vi "Client Single Connection.vi"() -> ()   [LabVIEW 2020]
doc: "This WebSockets API example VI acts as a client to make an outgoing websockets connection. Receives/sends string data to the connected server.\nWebSockets 2.0.1.40\nSam Sharp - MediaMongrels Ltd\nCopyright (c) 2019, MediaMongrels Ltd"
uses:
  Libraries/RPI.SenseHat.Joystick/TypeDefs/Joystick.ctl
  <vilib>/MediaMongrels Ltd/WebSockets/WebSockets/WebSocket/WebSocket.lvclass/WebSocket.ctl
  <vilib>/MediaMongrels Ltd/WebSockets/WebSockets/WebSocket Client/WebSocket Client.lvclass
  C:/Program Files (x86)/National Instruments/LabVIEW 2020/vi.lib/MediaMongrels Ltd/WebSockets/WebSockets/WebSocket/WebSocket.lvclass
  <vilib>/MediaMongrels Ltd/WebSockets/WebSockets/WebSocket/WebSocket.lvclass
  <vilib>/addons/_JKI.lib/Serialization/JSON/JKI JSON Serialization.lvlib
  Libraries/RPI.SenseHat.Joystick/RPI.SenseHat.Joystick.lvlib
panel:
  out "Joystick":T1
  in  "Send Id":bool
  in  "color 2":u32[][](array[colorbox])=[[16860, 16448250, 16711680, 0, 0, 0, 0, 0], [16860, 16448250, 16711680, 0, 0, 0, 0, 0], [16860, 16448250, 16711680, 0, 0, 0, 0, 0], [16777222, 0, 0, 0, 0, 0, 0, 0], [16777222, 0, 0, 0, 0, 0, 0, 0], [16777222, 0, 0, 0, 0, 0, 0, 0], [16777222, 0, 0, 0, 0, 0, 0, 0], [16777222, 0, 0, 0, 0, 0, 0, 0]] caption="Image"
  in  "draw":bool
  in  "fill":bool
  in  "clear":bool
  in  "reset":bool
  in  "color":u32(colorbox) caption="Color"
  in  "Disconnect":bool
  in  "Connect":bool
  in  "WebSockets URL":string="ws://192.168.0.27:6123"
  out "HTTP Headers":variant
  in  "Stop":bool
  out "Received Data":string
  in  "Send":bool
  in  "Data":string
  # "WebSockets Client Example"
  # "This VI is a simple example of sending/receiving data using WebSockets.\nIt opens a WebSockets Client connection to the WebSockets URL and can send / receive WebSockets data from the server.\n\nInstructions for use:\n1) Run this VI\n2) Enter the WebSockets URL that you wish to open a connection to (e.g. ws://echo.websocket.org) and click 'Connect'\n3) Enter text to send in 'Data' hit 'Send' to send to the WebSockets server\n4) WebSockets messages received from the server will be displayed in 'Received Data'"
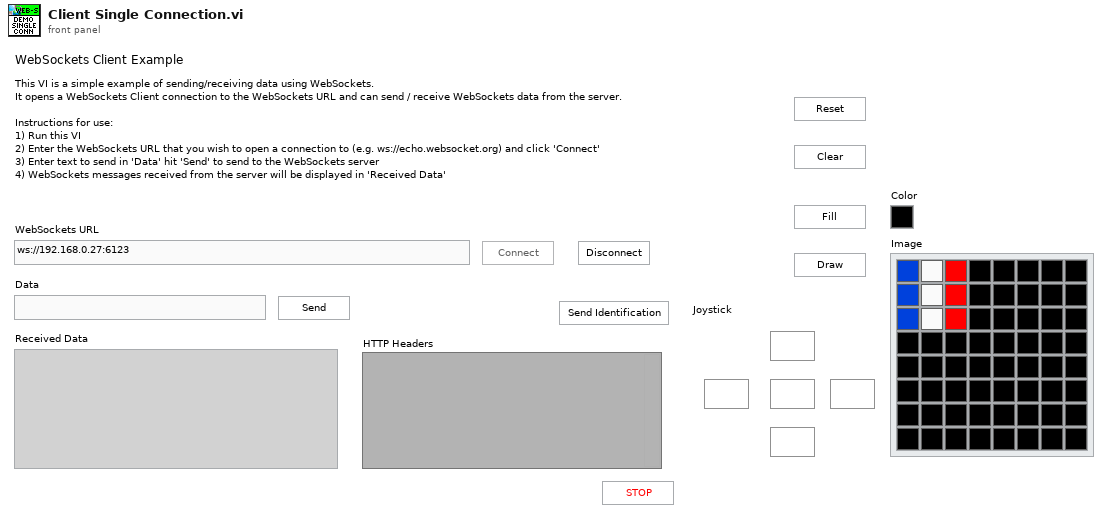
[diagram p1: front panel]
types:
  T1 = typedef "RPI.SenseHat.Joystick.lvlib/Joystick.ctl" = cluster{"Enter":bool, "Down":bool, "Up":bool, "Right":bool, "Left":bool}
  T2 = enum8{"Enabled", "Disabled", "Disabled and Grayed Out"}
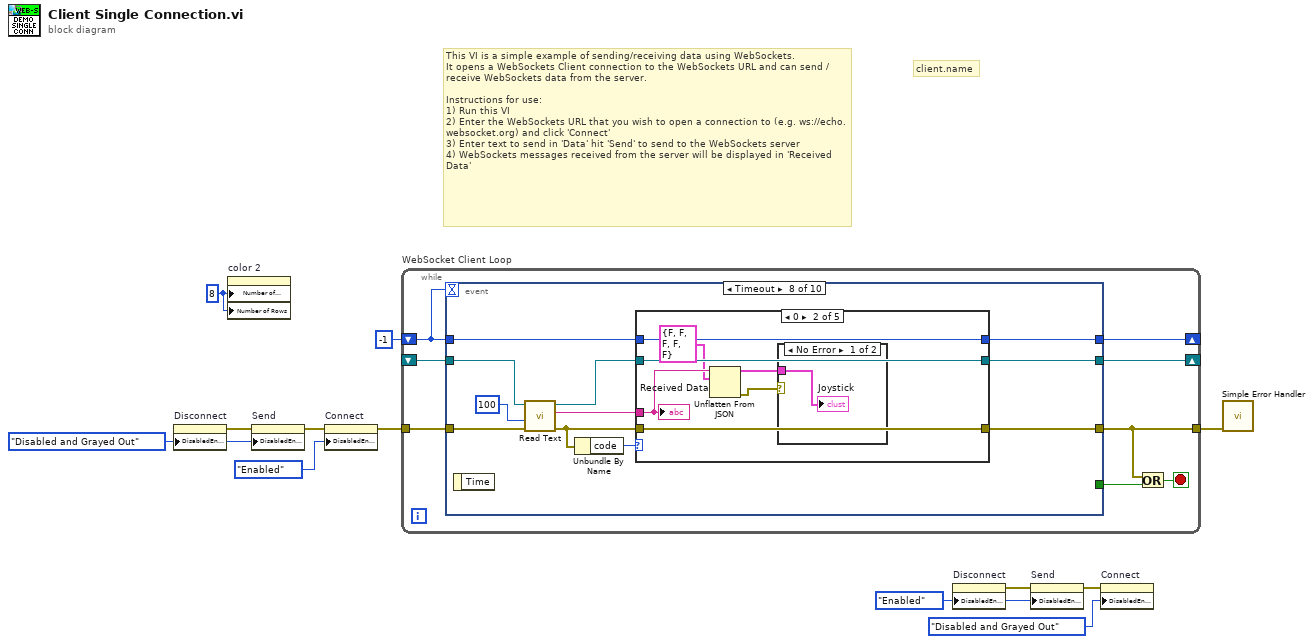
[diagram p0: block diagram]
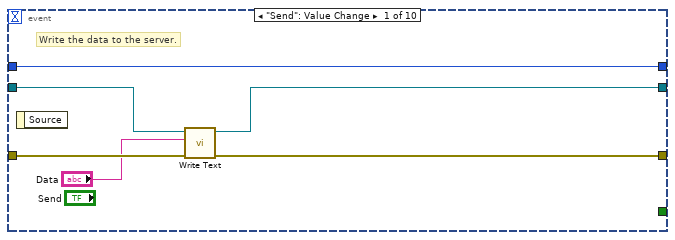
[diagram p2: hidden frame]
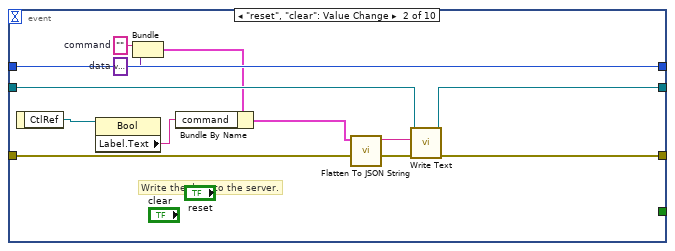
[diagram p3: hidden frame]
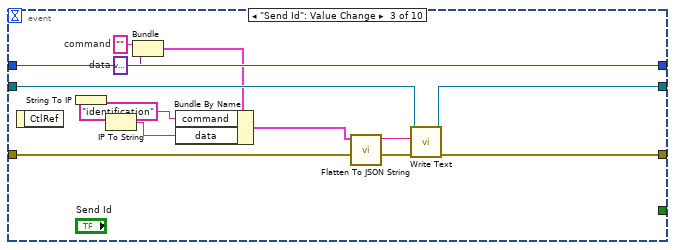
[diagram p4: hidden frame]
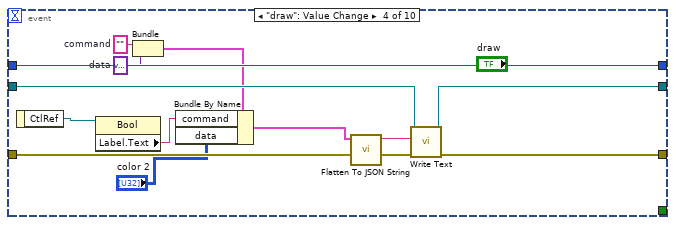
[diagram p5: hidden frame]
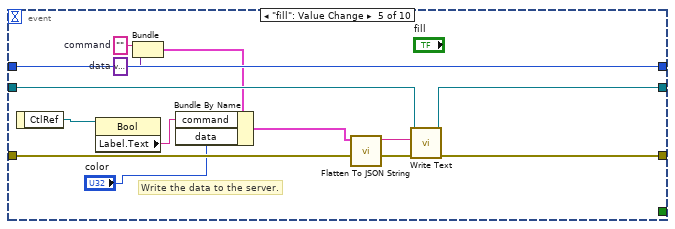
[diagram p6: hidden frame]
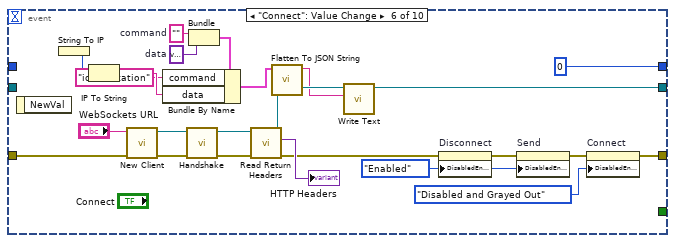
[diagram p7: hidden frame]
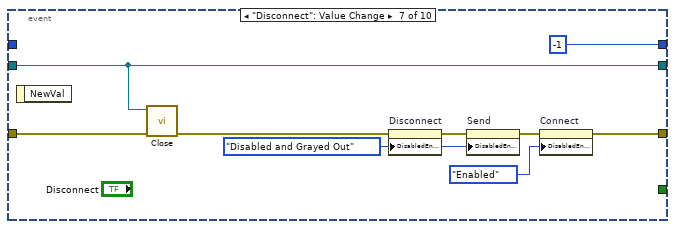
[diagram p8: hidden frame]
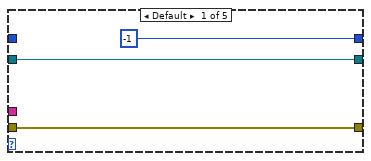
[diagram p9: hidden frame]
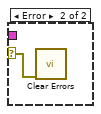
[diagram p10: hidden frame]
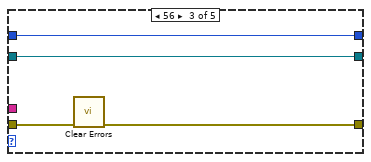
[diagram p11: hidden frame]
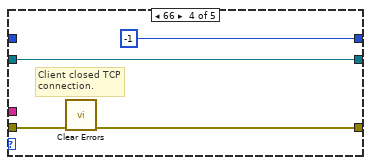
[diagram p12: hidden frame]
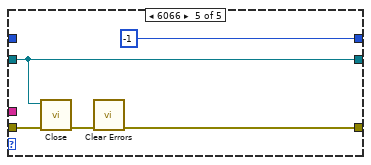
[diagram p13: hidden frame]
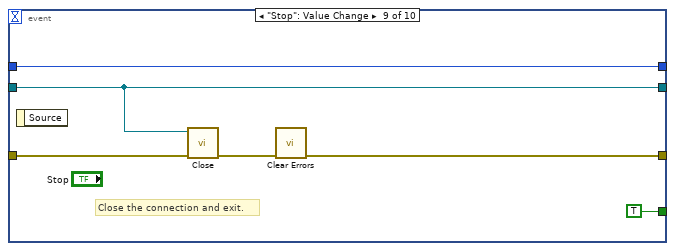
[diagram p14: hidden frame]
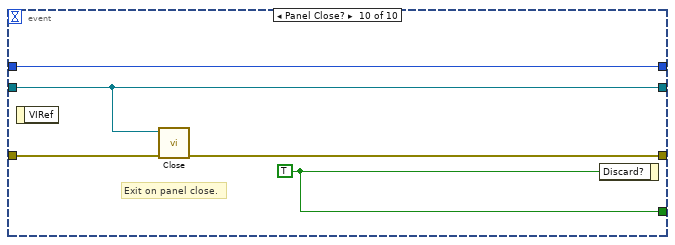
[diagram p15: hidden frame]
diagram:
  w1 = u32 8 ("Number of Columns")
  w5 = T2."Enabled" ("Disabled")
  w9 = T2."Disabled and Grayed Out" ("Disabled")
  # "client.name"
  # "This VI is a simple example of sending/receiving data using WebSockets.\nIt opens a WebSockets Client connection to the WebSockets URL and can send / receive WebSockets data from the server.\n\nInstructions for use:\n1) Run this VI\n2) Enter the WebSockets URL that you wish to open a connection to (e.g. ws://echo.websocket.org) and click 'Connect'\n3) Enter text to send in 'Data' hit 'Send' to send to the WebSockets server\n4) WebSockets messages received from the server will be displayed in 'Received Data'"
  n1 = property on="Disconnect" class="Bool"("DisabledEnum"=w9) -> (error out=w10:errorcluster)  [unwired: 2 in, 1 out]
  n2 = property on="color 2" class="Arr (strict)"("Number of Columns"=w1, "Number of Rows"=w1) -> ()  [unwired: 2 in, 2 out]
  n3 = property on="Send" class="Bool"(error in=w10, "DisabledEnum"=w9) -> (error out=w4:errorcluster)  [unwired: 1 in, 1 out]
  n4 = property on="Connect" class="Bool"(error in=w4, "DisabledEnum"=T2."Enabled" ("Disabled")) -> (error out=w3:errorcluster)  [unwired: 1 in, 1 out]
  n5 = while "WebSocket Client Loop" {
    tunnel: [w17] -> w12
    tunnel: w3 -> [w20]
    shift-right: [w16] -> _
    shift-left: _ -> [w15]
    shift-right: [w14] -> _
    shift-left: -1 -> [w13]
    stop <- w18 stop-if-true
    n6 = event shown="[7] Timeout" {
      selector: _ -> [_ _ _ _ _ _ _ _ _ _]
      dyn-events: _ -> [_ _ _ _ _ _ _ _ _ _]
      timeout: w13 -> [_ _ _ _ _ _ _ _ _ _]
      tunnel: [_ _ _ _ _ _ _ _ TRUE w157] -> w19
      tunnel: [w25 w37 w50 w63 w76 w88 w102 w116 w147 w155] -> w17
      tunnel: w20 -> [w26 w38 w51 w64 w77 w100 w110 w121 w151 w156]
      tunnel: [w22 w35 w48 w61 w74 w86 w109 w113 w149 w154] -> w16
      tunnel: w15 -> [w23 w36 w49 w62 w75 _ w109 w120 w149 w154]
      tunnel: w13 -> [w21 w34 w47 w60 w73 _ _ w112 w148 w153]
      tunnel: [w21 w34 w47 w60 w73 0 -1 w111 w148 w153] -> w14
      event "Send": Value Change {
        # "Write the data to the server."
        n7 = event-data() -> ()  [unwired: 1 in, 1 out]
        n8 = call-dynamic "Write Text.vi"("error in (no error)"=w26, "String Data"="Data", "WebSocket in"=w23) -> ("error out"=w25:errorcluster, "WebSocket out"=w22:refnum<class "WebSocket Client.lvclass">)  [unwired: 7 in]
      }
      event "reset", "clear": Value Change {
        w30 = variant  # data
        w31 = ""  # command
        # "Write the data to the server."
        n9 = event-data() -> ("CtlRef"=w32:refnum<vi>)  [unwired: 1 in]
        n10 = property class="Bool"(reference=w32) -> ("Label.Text"=w28:string)  [unwired: 1 in, 2 out]
        n11 = Bundle("command"=w31, "data"=w30) -> (w29:cluster{"command":string, "data":variant})  [unwired: 1 in]
        n12 = Bundle By Name(cluster=w29, "command"=w28) -> (w27:cluster{"command":string, "data":variant})
        n13 = call <vilib>:"Flatten To JSON String.vi"("Variant"=w27) -> ("JSON String"=w33:string)  [unwired: 9 in, 1 out]
        n14 = call-dynamic "Write Text.vi"("error in (no error)"=w38, "String Data"=w33, "WebSocket in"=w36) -> ("error out"=w37:errorcluster, "WebSocket out"=w35:refnum<class "WebSocket Client.lvclass">)  [unwired: 7 in]
      }
      event "Send Id": Value Change {
        w44 = variant  # data
        w45 = ""  # command
        n15 = event-data() -> ()  [unwired: 1 in, 1 out]
        n16 = String To IP() -> (0:w41:u32)  [unwired: 1 in]
        n17 = IP To String(2:w41) -> (0:w39:string)  [unwired: 1 in]
        n18 = Bundle("command"=w45, "data"=w44) -> (w43:cluster{"command":string, "data":variant})  [unwired: 1 in]
        n19 = Bundle By Name(cluster=w43, "command"="identification", "data"=w39) -> (w42:cluster{"command":string, "data":variant})
        n20 = call <vilib>:"Flatten To JSON String.vi"("Variant"=w42) -> ("JSON String"=w46:string)  [unwired: 9 in, 1 out]
        n21 = call-dynamic "Write Text.vi"("error in (no error)"=w51, "String Data"=w46, "WebSocket in"=w49) -> ("error out"=w50:errorcluster, "WebSocket out"=w48:refnum<class "WebSocket Client.lvclass">)  [unwired: 7 in]
      }
      event "draw": Value Change {
        w56 = variant  # data
        w57 = ""  # command
        n22 = event-data() -> ("CtlRef"=w58:refnum<vi>)  [unwired: 1 in]
        n23 = property class="Bool"(reference=w58) -> ("Label.Text"=w54:string)  [unwired: 1 in, 2 out]
        n24 = Bundle("command"=w57, "data"=w56) -> (w55:cluster{"command":string, "data":variant})  [unwired: 1 in]
        n25 = Bundle By Name(cluster=w55, "command"=w54, "data"="color 2") -> (w53:cluster{"command":string, "data":variant})
        n26 = call <vilib>:"Flatten To JSON String.vi"("Variant"=w53) -> ("JSON String"=w59:string)  [unwired: 9 in, 1 out]
        n27 = call-dynamic "Write Text.vi"("error in (no error)"=w64, "String Data"=w59, "WebSocket in"=w62) -> ("error out"=w63:errorcluster, "WebSocket out"=w61:refnum<class "WebSocket Client.lvclass">)  [unwired: 7 in]
      }
      event "fill": Value Change {
        w69 = variant  # data
        w70 = ""  # command
        # "Write the data to the server."
        n28 = event-data() -> ("CtlRef"=w71:refnum<vi>)  [unwired: 1 in]
        n29 = property class="Bool"(reference=w71) -> ("Label.Text"=w67:string)  [unwired: 1 in, 2 out]
        n30 = Bundle("command"=w70, "data"=w69) -> (w68:cluster{"command":string, "data":variant})  [unwired: 1 in]
        n31 = Bundle By Name(cluster=w68, "command"=w67, "data"="color") -> (w66:cluster{"command":string, "data":variant})
        n32 = call <vilib>:"Flatten To JSON String.vi"("Variant"=w66) -> ("JSON String"=w72:string)  [unwired: 9 in, 1 out]
        n33 = call-dynamic "Write Text.vi"("error in (no error)"=w77, "String Data"=w72, "WebSocket in"=w75) -> ("error out"=w76:errorcluster, "WebSocket out"=w74:refnum<class "WebSocket Client.lvclass">)  [unwired: 7 in]
      }
      event "Connect": Value Change {
        w83 = variant  # data
        w84 = ""  # command
        w92 = T2."Enabled" ("Disabled")
        n34 = event-data() -> ()  [unwired: 1 in, 1 out]
        n35 = String To IP() -> (0:w85:u32)  [unwired: 1 in]
        n36 = IP To String(2:w85) -> (0:w81:string)  [unwired: 1 in]
        n37 = call <vilib>:"New Client.vi"("error in (no error)"=w100, "WebSocket URL"="WebSockets URL") -> ("error out"=w101:errorcluster, "WebSocket Client out"=w98:refnum<class "WebSocket Client.lvclass">)  [unwired: 8 in]
        n38 = call-dynamic "Handshake.vi"("error in (no error)"=w101, "WebSocket Client in"=w98) -> ("error out"=w97:errorcluster, "WebSocket Client out"=w96:refnum<class "WebSocket Client.lvclass">)  [unwired: 8 in]
        n39 = Bundle("command"=w84, "data"=w83) -> (w82:cluster{"command":string, "data":variant})  [unwired: 1 in]
        n40 = Bundle By Name(cluster=w82, "command"="identification", "data"=w81) -> (w79:cluster{"command":string, "data":variant})
        n41 = call <vilib>:"Read Return Headers.vi"("error in (no error)"=w97, "WebSocket in"=w96) -> ("error out"=w90:errorcluster, "Return Headers"=→"HTTP Headers":variant, "WebSocket out"=w95:refnum<class "WebSocket Client.lvclass">)  [unwired: 7 in]
        n42 = call <vilib>:"Flatten To JSON String.vi"("Variant"=w79) -> ("JSON String"=w78:string)  [unwired: 9 in, 1 out]
        n43 = call-dynamic "Write Text.vi"("String Data"=w78, "WebSocket in"=w95) -> ("WebSocket out"=w86:refnum<class "WebSocket Client.lvclass">)  [unwired: 8 in, 1 out]
        n44 = property on="Disconnect" class="Bool"(error in=w90, "DisabledEnum"=w92) -> (error out=w91:errorcluster)  [unwired: 1 in, 1 out]
        n45 = property on="Send" class="Bool"(error in=w91, "DisabledEnum"=w92) -> (error out=w89:errorcluster)  [unwired: 1 in, 1 out]
        n46 = property on="Connect" class="Bool"(error in=w89, "DisabledEnum"=T2."Disabled and Grayed Out" ("Disabled")) -> (error out=w88:errorcluster)  [unwired: 1 in, 1 out]
      }
      event "Disconnect": Value Change {
        w105 = T2."Disabled and Grayed Out" ("Disabled")
        n47 = event-data() -> ()  [unwired: 1 in, 1 out]
        n48 = call-dynamic "Close.vi"("error in (no error)"=w110, "WebSocket in"=w109) -> ("error out"=w103:errorcluster)  [unwired: 9 in]
        n49 = property on="Disconnect" class="Bool"(error in=w103, "DisabledEnum"=w105) -> (error out=w104:errorcluster)  [unwired: 1 in, 1 out]
        n50 = property on="Send" class="Bool"(error in=w104, "DisabledEnum"=w105) -> (error out=w106:errorcluster)  [unwired: 1 in, 1 out]
        n51 = property on="Connect" class="Bool"(error in=w106, "DisabledEnum"=T2."Enabled" ("Disabled")) -> (error out=w102:errorcluster)  [unwired: 1 in, 1 out]
      }
      event Timeout {
        n52 = event-data() -> ()  [unwired: 1 in, 1 out]
        n53 = call-dynamic "Read Text.vi"("error in (no error)"=w121, "timeout ms (5000)"=100, "WebSocket in"=w120) -> ("error out"=w115:errorcluster, "Data"=w118:string, "WebSocket out"=w114:refnum<class "WebSocket Client.lvclass">)  [unwired: 6 in]
        n54 = Unbundle By Name(w115) -> ("code"=w117:i32)
        n55 = case shown="0" w117 {
          tunnel: w118 -> [_ w128 _ _ _]
          tunnel: [w124 w131 w136 w138 w142] -> w116
          tunnel: w115 -> [w124 w131 w137 w141 w146]
          tunnel: w114 -> [w123 w130 w135 w140 w144]
          tunnel: [w123 w130 w135 w140 w144] -> w113
          tunnel: w112 -> [_ w129 w134 _ _]
          tunnel: [-1 w129 w134 -1 -1] -> w111
          frame Default {
          }
          frame 0 {
            n56 = Unflatten From JSON(JSON string=w128, type and defaults=T1 {"Enter"=FALSE, "Down"=FALSE, "Up"=FALSE, "Right"=FALSE, "Left"=FALSE} ("Joystick")) -> (value=w125:T1, error out=w126:errorcluster)  [unwired: 5 in]
            n57 = case shown="No Error" w126 {
              selector: w126 -> [_ w133]
              tunnel: w125 -> [w132 _]
              frame No Error {
                "Joystick" <- w132
              }
              frame Error {
                n58 = call <vilib>:"Clear Errors.vi"("error in (no error)"=w133) -> ()  [unwired: 5 in, 2 out]
              }
            }
            "Received Data" <- w128
          }
          frame 56 {
            n59 = call <vilib>:"Clear Errors.vi"("error in (no error)"=w137) -> ("error out"=w136:errorcluster)  [unwired: 5 in, 1 out]
          }
          frame 66 {
            # "Client closed TCP connection."
            n60 = call <vilib>:"Clear Errors.vi"("error in (no error)"=w141) -> ("error out"=w138:errorcluster)  [unwired: 5 in, 1 out]
          }
          frame 6066 {
            n61 = call-dynamic "Close.vi"("error in (no error)"=w146, "WebSocket in"=w144) -> ("error out"=w145:errorcluster)  [unwired: 9 in]
            n62 = call <vilib>:"Clear Errors.vi"("error in (no error)"=w145) -> ("error out"=w142:errorcluster)  [unwired: 5 in, 1 out]
          }
        }
      }
      event "Stop": Value Change {
        # "Close the connection and exit."
        n63 = event-data() -> ()  [unwired: 1 in, 1 out]
        n64 = call-dynamic "Close.vi"("error in (no error)"=w151, "WebSocket in"=w149) -> ("error out"=w150:errorcluster)  [unwired: 9 in]
        n65 = call <vilib>:"Clear Errors.vi"("error in (no error)"=w150) -> ("error out"=w147:errorcluster)  [unwired: 5 in, 1 out]
      }
      event Panel Close? {
        w157 = TRUE ("Discard?")
        # "Exit on panel close."
        n66 = event-data() -> ()  [unwired: 1 in, 1 out]
        n67 = call-dynamic "Close.vi"("error in (no error)"=w156, "WebSocket in"=w154) -> ("error out"=w155:errorcluster)  [unwired: 9 in]
        n68 = event-data("Discard?"=w157) -> ()  [unwired: 1 in, 1 out]
      }
    }
    n69 = Or(x=w17, y=w19) -> (x .or. y?=w18:bool)
  }
  n70 = property on="Disconnect" class="Bool"("DisabledEnum"=w5) -> (error out=w6:errorcluster)  [unwired: 2 in, 1 out]
  n71 = property on="Send" class="Bool"(error in=w6, "DisabledEnum"=w5) -> (error out=w7:errorcluster)  [unwired: 1 in, 1 out]
  n72 = property on="Connect" class="Bool"(error in=w7, "DisabledEnum"=T2."Disabled and Grayed Out" ("Disabled")) -> ()  [unwired: 1 in, 2 out]
  n73 = call <vilib>:"Simple Error Handler.vi"("error in (no error)"=w12) -> ()  [unwired: 4 in, 5 out]
